vi "RSZVB Select Calibration Type.vi"(0 "VISA session":refnum<visa-resource-name>, 1 "Port 2 (1)":i32=1, 2 "Port 1 (1)":i32=1, 5 "Channel (1)":i32=1, 7 "Calibration Name":string, 9 "Parameters (0: One-port Normalization (reflection, open standard))":i32(ring) items=["One-port Normalization (reflection, open standard)"=0, "One-port Normalization (reflection, short standard)"=1, "Full One Port"=2, "Two-port Normalization"=3, "One Path Two Port"=4, "TOSM"=5, "TOM"=6, "TRM"=7, "TRL"=8, "TNA"=9, "TOSM With Unknown Through"=12, "Forward Transmission"=13, "Backward Transmission"=14, "NIST Multiline TRL"=16], 11 "error in (no error)":errorcluster {"code" format="%.0x"}, 12 "Port 3 (1)":i32=1, 13 "Port 4 (1)":i32=1) -> (4 "dup VISA session":refnum<visa-resource-name>, 15 "error out":errorcluster {"code" format="%.0x"})   [LabVIEW 2011]
doc: "This VI selects a one-port, two-port, three-port or four-port calibration type at arbitrary analyzer ports.\n\nNote(s):\n\n(1) For an n-port calibration type (n = 1 to 4), n port numbers must be specified. If more than n numbers are defined, the spare numbers (the last in the list) are ignored.\n\nRemote-control command(s):\n[SENSe<Ch>:]CORRection:COLLect:METHod:DEFine '<cal_name>', REFL | RSHort | FOPort | FRTRans | OPTPort | TOSM | TOM | TRM | TRL | TNA, <port_no>[,<port_no>][,<port_no>][,<port_no>]"
uses:
  _utility/RSZVB Global Data.vi
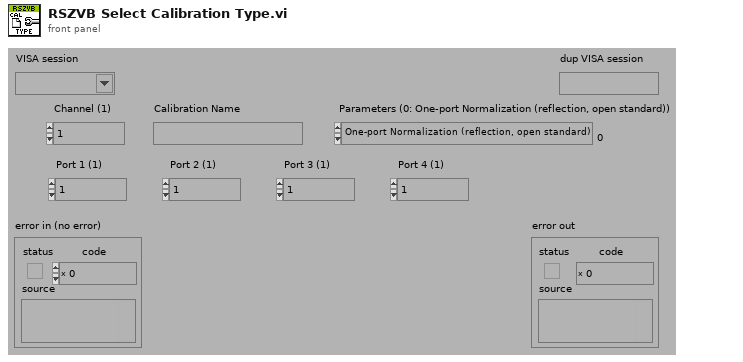
[diagram p1: front panel]
types:
  T1 = cluster{"Error Checking (T: On)":bool, "Installed Options":string[], "Data Valid?":bool, "Ports":i32, "Model":string[], "Option Checking (T: On)":bool}[]
  T2 = cluster{"Error Checking (T: On)":bool, "Installed Options":string[], "Data Valid?":bool, "Ports":i32, "Model":string[], "Option Checking (T: On)":bool}
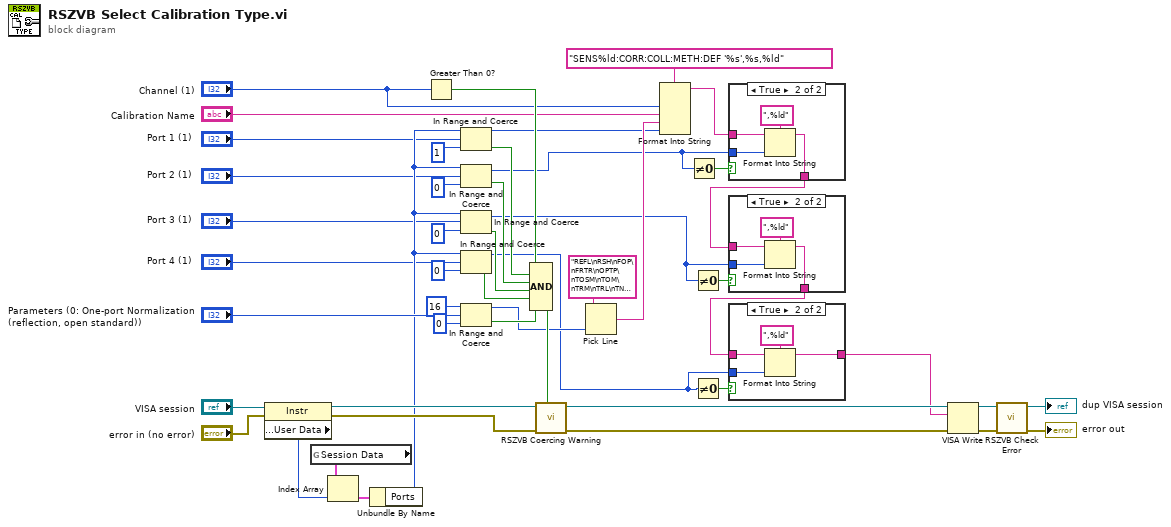
[diagram p0: block diagram]
diagram:
  n1 = property class="Instr"(reference="VISA session", error in="error in (no error)") -> (reference out=w38:refnum<visa-resource-name>, error out=w39:errorcluster, "General Settings:User Data"=w40:u32)
  n2 = global read "RSZVB Global Data.vi" "Session Data"() -> (w41:T1)
  n3 = Index Array(array=w41, index=w40) -> (element=w42:T2)
  n4 = Unbundle By Name(w42) -> ("Ports"=w24:i32)
  n5 = Greater Than 0?(x="Channel (1)") -> (x > 0?=w43:bool)
  n6 = In Range and Coerce(upper limit=w24, x="Port 1 (1)", lower limit=1) -> (coerced(x)=w18:i32, In Range?=w17:bool)
  n7 = In Range and Coerce(upper limit=w24, x="Port 2 (1)", lower limit=0) -> (coerced(x)=w8:i32, In Range?=w16:bool)
  n8 = In Range and Coerce(upper limit=w24, x="Port 3 (1)", lower limit=0) -> (coerced(x)=w6:i32, In Range?=w15:bool)
  n9 = In Range and Coerce(upper limit=w24, x="Port 4 (1)", lower limit=0) -> (coerced(x)=w3:i32, In Range?=w14:bool)
  n10 = In Range and Coerce(upper limit=16 ("lower limit"), x="Parameters (0: One-port Normalization (reflection, open standard))", lower limit=0) -> (coerced(x)=w12:i32, In Range?=w13:bool)
  n11 = Compound Arithmetic op=AND(w43, w17, w16, w15, w14, w13) -> (w44:bool)
  n12 = call "RSZVB Coercing Warning.vi"("In Range?"=w44, "error in (no error)"=w39, "VISA session"=w38) -> ("error out"=w47:errorcluster, "dup VISA session"=w48:refnum<visa-resource-name>)  [unwired: 7 in]
  n13 = Pick Line(multi-line string="REFL\nRSH\nFOP\nFRTR\nOPTP\nTOSM\nTOM\nTRM\nTRL\nTNA\nFNP\nSFTP\nUOSM\nFTR\nRTR\nOSM\nNMTR", line index=w12) -> (output string=w34:string)  [unwired: 1 in]
  n14 = Format Into String(format string="SENS%ld:CORR:COLL:METH:DEF '%s',%s,%ld", "Channel (1)", "Calibration Name", w34, w18) -> (resulting string=w9:string)  [unwired: 2 in, 1 out]
  n15 = Not Equal To 0?(x=w8) -> (x != 0?=w10:bool)
  n16 = Not Equal To 0?(x=w6) -> (x != 0?=w7:bool)
  n17 = Not Equal To 0?(x=w3) -> (x != 0?=w4:bool)
  n18 = case shown="True" w10 {
    tunnel: w9 -> [w50 w54]
    tunnel: w8 -> [_ w52]
    tunnel: [w50 w51] -> w5
    frame False {
    }
    frame True {
      n19 = Format Into String(format string=",%ld", initial string=w54, w52) -> (resulting string=w51:string)  [unwired: 1 in, 1 out]
    }
  }
  n20 = case shown="True" w7 {
    tunnel: w5 -> [w55 w59]
    tunnel: w6 -> [_ w57]
    tunnel: [w55 w56] -> w2
    frame False {
    }
    frame True {
      n21 = Format Into String(format string=",%ld", initial string=w59, w57) -> (resulting string=w56:string)  [unwired: 1 in, 1 out]
    }
  }
  n22 = case shown="True" w4 {
    tunnel: w2 -> [w60 w64]
    tunnel: w3 -> [_ w62]
    tunnel: [w60 w61] -> w1
    frame False {
    }
    frame True {
      n23 = Format Into String(format string=",%ld", initial string=w64, w62) -> (resulting string=w61:string)  [unwired: 1 in, 1 out]
    }
  }
  n24 = VISA Write(VISA resource name=w48, write buffer=w1, error in (no error)=w47) -> (VISA resource name out=w45:refnum<visa-resource-name>, error out=w46:errorcluster)  [unwired: 1 out]
  n25 = call "RSZVB Check Error.vi"("error in (no error)"=w46, "VISA session"=w45) -> ("error out"=→"error out":errorcluster, "dup VISA session"=→"dup VISA session":refnum<visa-resource-name>)  [unwired: 8 in]
